vi "VLC Test VI.vi"   [LabVIEW 2020, in "VLC Wrapper.lvclass"]
uses:
  VLC Wrapper.lvclass
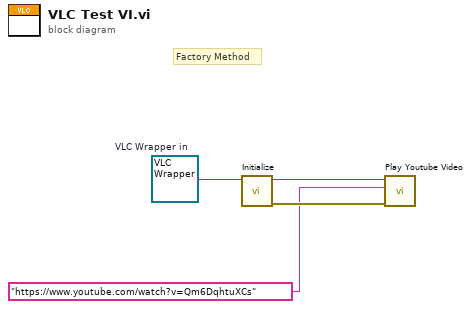
[diagram p0: block diagram]
diagram:
  w2 = refnum<class "VLC Wrapper.lvclass"> refnum  # VLC Wrapper in
  # "Factory Method"
  n1 = call-dynamic "Initialize.vi"("VLC Wrapper in"=w2) -> ("error out"=w3:errorcluster, "VLC Wrapper out"=w4:refnum<class "VLC Wrapper.lvclass">)  [unwired: 9 in]
  n2 = call "Play Youtube Video.vi"("error in (no error)"=w3, "Youtube URL"="https://www.youtube.com/watch?v=Qm6DqhtuXCs" ("Youtupe URL"), "VLC Wrapper in"=w4) -> ()  [unwired: 7 in, 2 out]
